vi "Read A Theme is Loaded.vi"(8 "error in (no error)":errorcluster, 11 "Generic Theme in":refnum<class "Generic Theme.lvclass">) -> (0 "error out":errorcluster, 2 "A Theme is Loaded":bool, 3 "Generic Theme out":refnum<class "Generic Theme.lvclass">)   [LabVIEW 2021, in "Appearance Actor.lvlib" / "Generic Theme.lvclass"]
uses:
  Generic Theme.lvclass
  Generic Theme.lvclass/Generic Theme.ctl
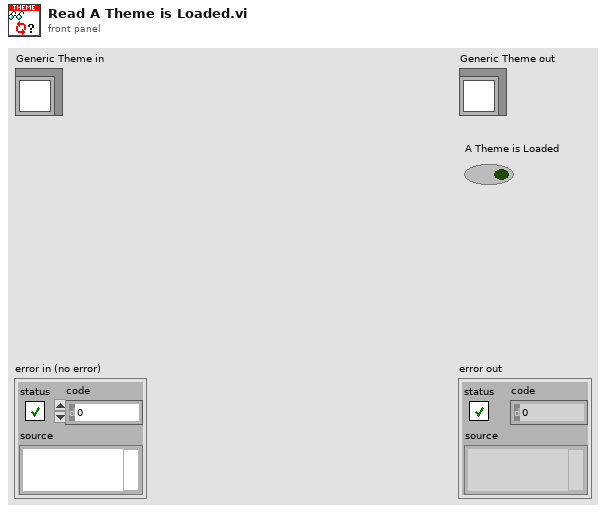
[diagram p1: front panel]
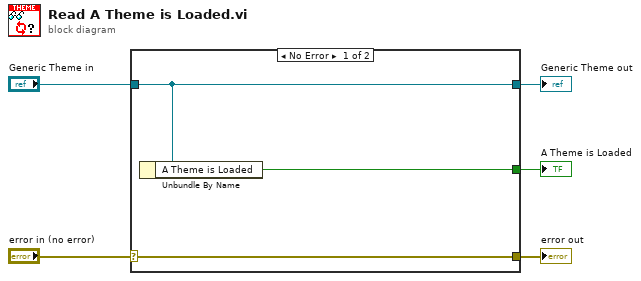
[diagram p0: block diagram]
diagram:
  n1 = case shown="No Error" "error in (no error)" {
    selector: "error in (no error)" -> [w8 w9]
    tunnel: [w8 w9] -> w4
    tunnel: [w7 w10] -> w2
    tunnel: "Generic Theme in" -> [w7 w10]
    tunnel: [w6 _] -> w1
    frame No Error {
      n2 = Unbundle By Name(w7) -> ("A Theme is Loaded"=w6:bool)
    }
    frame Error {
    }
  }
  "error out" <- w4
  "Generic Theme out" <- w2
  "A Theme is Loaded" <- w1
